vi "VISA-TEST.vi"(10 "Tx":u8[](array[numeric]), 11 "VISA":refnum<visa-resource-name>) -> (1 "good?":bool, 2 "Rx":u8[](array[numeric]), 3 "VISA":refnum<visa-resource-name>)   [LabVIEW 2018]
panel:
  out "read buffer 2":string
  out "null？":bool
  out "read buffer":string
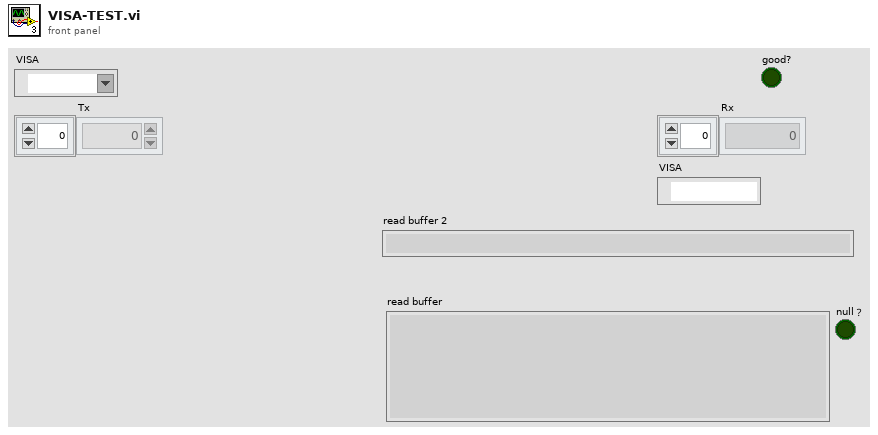
[diagram p1: front panel]
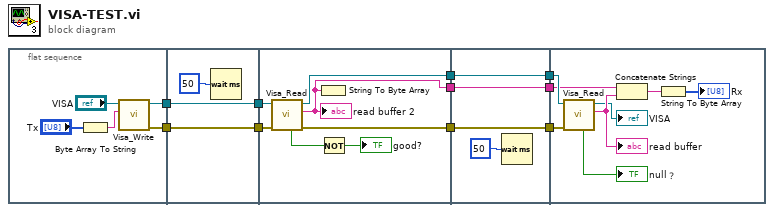
[diagram p0: block diagram]
diagram:
  n1 = flat-sequence {
    tunnel: [w14] -> w10
    tunnel: [w13] -> w8
    tunnel: w10 -> [w17]
    tunnel: [w17] -> w9
    tunnel: w8 -> [w16]
    tunnel: [w16] -> w7
    tunnel: w9 -> [w25]
    tunnel: w7 -> [w24]
    tunnel: [w22] -> w6
    tunnel: [w21] -> w4
    tunnel: [w20] -> w2
    tunnel: w6 -> [w29]
    tunnel: [w29] -> w5
    tunnel: w4 -> [w28]
    tunnel: [w28] -> w3
    tunnel: w2 -> [w27]
    tunnel: [w27] -> w1
    tunnel: w5 -> [w37]
    tunnel: w3 -> [w36]
    tunnel: w1 -> [w34]
    frame #0 {
      n2 = Byte Array To String(unsigned byte array="Tx") -> (string=w12:string)
      n3 = call "Visa_Write.vi"("write"=w12, "VISA"="VISA") -> ("错误输出"=w13:errorcluster, "VISA"=w14:refnum<visa-resource-name>)  [unwired: 8 in]
    }
    frame #1 {
      n4 = Wait (ms)(milliseconds to wait=u32 50 ("等待时间（毫秒）")) -> ()  [unwired: 1 out]
    }
    frame #2 {
      n5 = call "Visa_Read.vi"("错误输入（无错误）"=w24, "VISA"=w25) -> ("error out"=w21:errorcluster, "read buffer"=w20:string, "VISA"=w22:refnum<visa-resource-name>, "null？"=w19:bool)  [unwired: 5 in, 1 out]
      "read buffer 2" <- w20
      n6 = String To Byte Array(string=w20) -> ()  [unwired: 1 out]
      n7 = Not(x=w19) -> (.not. x?=→"good?":bool)
    }
    frame #3 {
      n8 = Wait (ms)(milliseconds to wait=u32 50 ("等待时间（毫秒）")) -> ()  [unwired: 1 out]
    }
    frame #4 {
      n9 = call "Visa_Read.vi"("错误输入（无错误）"=w36, "VISA"=w37) -> ("read buffer"=w33:string, "VISA"=→"VISA":refnum<visa-resource-name>, "null？"=→"null？":bool)  [unwired: 5 in, 2 out]
      "read buffer" <- w33
      n10 = Concatenate Strings(w34, w33) -> (w32:string)
      n11 = String To Byte Array(string=w32) -> (unsigned byte array=→"Rx":u8[])
    }
  }
